vi "Write Multiple Holding Registers.vi"(8 "error in (no error)":errorcluster, 9 "holding register values":u16[](array[numeric]), 10 "starting address":u16, 11 "Modbus master in":refnum<class "Modbus Master.lvclass">) -> (0 "error out":errorcluster, 3 "Modbus master out":refnum<class "Modbus Master.lvclass">)   [LabVIEW 2021, in "Modbus Master.lvclass"]
doc: "Writes values to contiguous holding registers. The maximum number of holding registers this VI can write is 123."
uses:
  Modbus Master.lvclass
  Modbus Master.lvclass/Modbus Master.ctl
  Network Protocol/Network Master/Network Master.lvclass
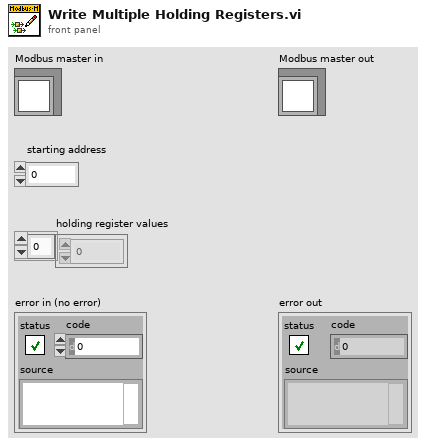
[diagram p1: front panel]
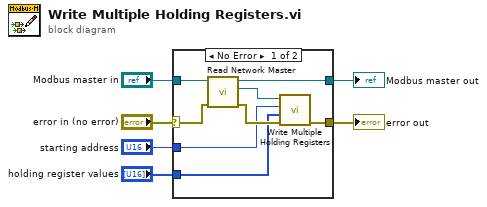
[diagram p0: block diagram]
diagram:
  n1 = case shown="No Error" "error in (no error)" {
    selector: "error in (no error)" -> [w12 w16]
    tunnel: "Modbus master in" -> [w13 w15]
    tunnel: [w9 w16] -> w3
    tunnel: [w14 w15] -> w4
    tunnel: "holding register values" -> [w7 _]
    tunnel: "starting address" -> [w8 _]
    frame No Error {
      n2 = call "Read Network Master.vi"("error in"=w12, "Modbus master in"=w13) -> ("error out"=w10:errorcluster, "Network Master"=w11:refnum<class "Network Master.lvclass">, "Modbus master out"=w14:refnum<class "Modbus Master.lvclass">)  [unwired: 7 in]
      n3 = call "Write Multiple Holding Registers.vi"("error in (no error)"=w10, "holding register values"=w7, "starting address"=w8, "Modbus master in"=w11) -> ("error out"=w9:errorcluster)  [unwired: 6 in, 1 out]
    }
    frame Error {
    }
  }
  "error out" <- w3
  "Modbus master out" <- w4
